vi "Pop.vi"(11 "Stack in":refnum<class "Stack.lvclass">) -> (1 "Popped Payload":variant, 2 "Popped Action":string, 3 "Stack out":refnum<class "Stack.lvclass">)   [LabVIEW 2024, in "ActionStack.lvlib" / "Stack.lvclass"]
uses:
  Stack.lvclass
  Stack.lvclass/Stack.ctl
  Action/Action.lvclass
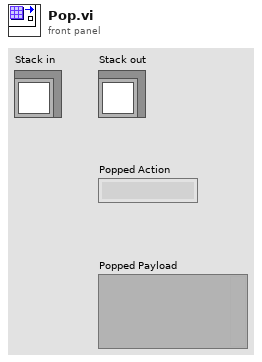
[diagram p1: front panel]
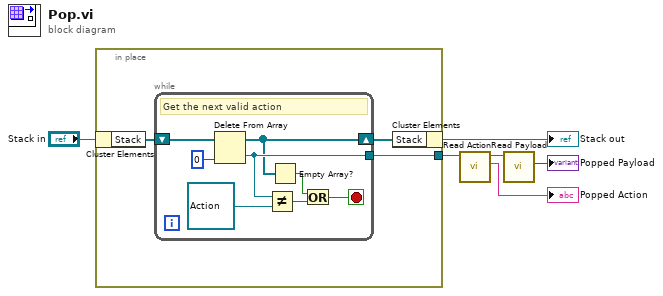
[diagram p0: block diagram]
diagram:
  n1 = in-place {
    in-place-border: [w9] -> w3
    n2 = in-place-cluster #1("Stack in") -> ("Stack"=w8:refnum<class "Action.lvclass">[])
    n3 = while {
      tunnel: [w15] -> w9
      shift-right: [w14] -> w7
      shift-left: w8 -> [w17]
      stop <- w11 stop-if-true
      # "Get the next valid action"
      n4 = Delete From Array(array=w17, index=0) -> (deleted portion=w15:refnum<class "Action.lvclass">, array with subset deleted=w14:refnum<class "Action.lvclass">[])  [unwired: 1 in]
      n5 = Not Equal?(x=w15, y=refnum<class "Action.lvclass"> refnum ("Action.lvclass")) -> (x != y?=w12:bool)
      n6 = Empty Array?(array=w14) -> (empty?=w13:bool)
      n7 = Or(x=w13, y=w12) -> (x .or. y?=w11:bool)
    }
    n8 = in-place-cluster #1("Stack"=w7) -> (→"Stack out":refnum<class "Stack.lvclass">)
  }
  n9 = call "Read Action.vi"("ActionStack in"=w3) -> ("Action"=→"Popped Action":string, "ActionStack out"=w6:refnum<class "Action.lvclass">)  [unwired: 9 in]
  n10 = call "Read Payload.vi"("ActionStack in"=w6) -> ("Payload"=→"Popped Payload":variant)  [unwired: 9 in, 1 out]
